vi "Calculate Quasi Peak Voltage Factor.vi"(9 "Charging":bool, 10 "Time Constant":dbl format="%#_13g", 11 "Sample Rate":dbl format="%#_13g") -> (2 "Voltage Factor":dbl format="%#_12g")   [LabVIEW 2017]
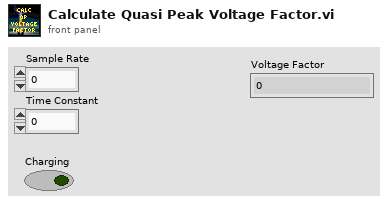
[diagram p1: front panel]
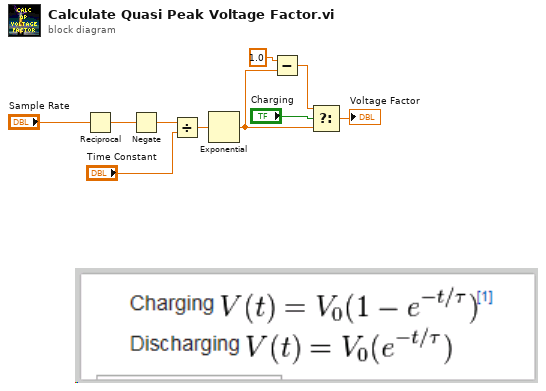
[diagram p0: block diagram]
diagram:
  n1 = Reciprocal(x="Sample Rate") -> (1/x=w8:dbl)
  n2 = Negate(x=w8) -> (-x=w7:dbl)
  n3 = Divide(x=w7, y="Time Constant") -> (x/y=w5:dbl)
  n4 = Exponential(1:w5) -> (0:w3:dbl)
  n5 = Subtract(x=1.0, y=w3) -> (x-y=w2:dbl)
  n6 = Select(t=w2, s="Charging", f=w3) -> (s? t:f=→"Voltage Factor":dbl)
